vi "NewDoor.vi"(8 "error in (no error)":errorcluster, 10 "Room 2":refnum<class "Room.lvclass">, 11 "Room 1":refnum<class "Room.lvclass">) -> (0 "error out":errorcluster, 3 "Door":refnum<class "Door.lvclass">)   [LabVIEW 2020, in "Door.lvclass"]
uses:
  Door.lvclass
  Room/Room.lvclass
  Door.lvclass/Door.ctl
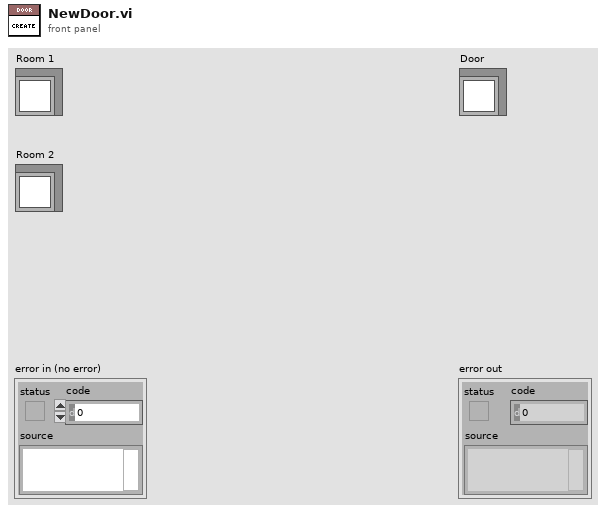
[diagram p1: front panel]
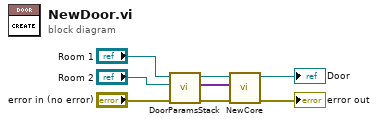
[diagram p0: block diagram]
diagram:
  n1 = call "DoorParamsStack.vi"("error in (no error)"="error in (no error)", "room2"="Room 2", "room1"="Room 1") -> ("error out"=w8:errorcluster, "HierarchyParams"=w7:variant[], "Door"=w6:refnum<class "Door.lvclass">)  [unwired: 6 in]
  n2 = call-dynamic "NewCore.vi"("error in (no error)"=w8, "ParamsArray"=w7, "Door"=w6) -> ("error out"=→"error out":errorcluster, "Door"=→"Door":refnum<class "Door.lvclass">)  [unwired: 7 in]
